vi "Set count lmits.vi"(8 "error in (no error)":errorcluster, 9 "Production max limit":dbl, 10 "Reel max limit":dbl, 11 "Counts":refnum<vi>) -> (0 "error out":errorcluster)   [LabVIEW 2019, in "ZenGage v3.0 UI.lvclass"]
uses:
  ZenGage v3.0 UI.lvclass
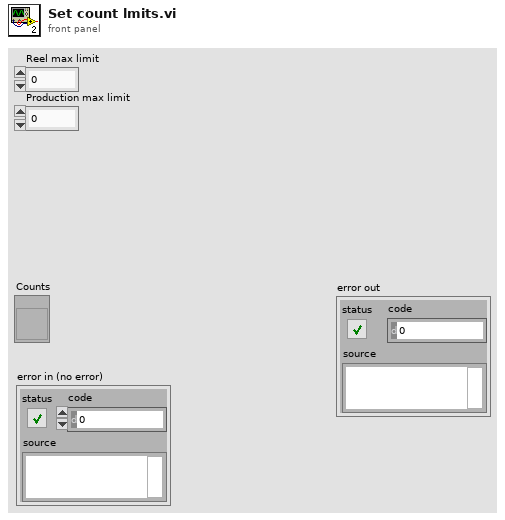
[diagram p1: front panel]
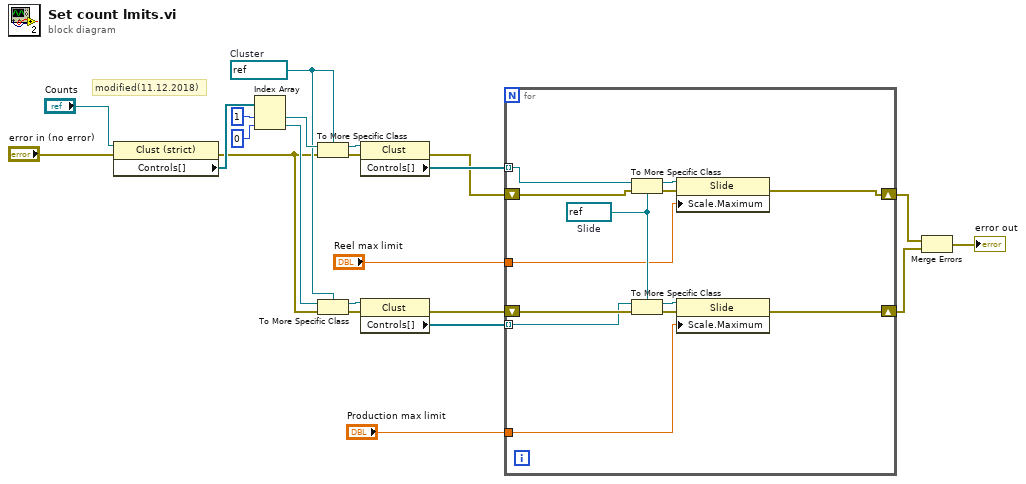
[diagram p0: block diagram]
diagram:
  w15 = refnum<vi> refnum  # Cluster
  # "modified(11.12.2018)"
  n1 = property class="Clust (strict)"(reference="Counts", error in="error in (no error)") -> (error out=w9:errorcluster, "Controls[]"=w22:refnum<vi>[])  [unwired: 1 out]
  n2 = Index Array(array=w22, index #1=1 ("index"), index #2=0 ("index")) -> (element #1=w19:refnum<vi>, element #2=w16:refnum<vi>)
  n3 = To More Specific Class(target class=w15, reference=w19, error in=w9) -> (specific class reference=w18:refnum<vi>, error out=w8:errorcluster)
  n4 = To More Specific Class(target class=w15, reference=w16, error in=w9) -> (specific class reference=w14:refnum<vi>, error out=w7:errorcluster)
  n5 = property class="Clust"(reference=w18, error in=w8) -> (error out=w6:errorcluster, "Controls[]"=w17:refnum<vi>[])  [unwired: 1 out]
  n6 = property class="Clust"(reference=w14, error in=w7) -> (error out=w5:errorcluster, "Controls[]"=w13:refnum<vi>[])  [unwired: 1 out]
  n7 = for {
    tunnel: w17 -> [w24] mode=indexing
    tunnel: w13 -> [w23] mode=indexing
    tunnel: "Reel max limit" -> [w32]
    tunnel: "Production max limit" -> [w31]
    shift-right: [w26] -> w2
    shift-left: w6 -> [w30]
    shift-right: [w25] -> w3
    shift-left: w5 -> [w29]
    w33 = refnum<vi> refnum  # Slide
    n8 = To More Specific Class(target class=w33, reference=w24, error in=w30) -> (specific class reference=w35:refnum<vi>, error out=w28:errorcluster)
    n9 = To More Specific Class(target class=w33, reference=w23, error in=w29) -> (specific class reference=w34:refnum<vi>, error out=w27:errorcluster)
    n10 = property class="Slide"(reference=w35, error in=w28, "Scale.Maximum"=w32) -> (error out=w26:errorcluster)  [unwired: 1 out]
    n11 = property class="Slide"(reference=w34, error in=w27, "Scale.Maximum"=w31) -> (error out=w25:errorcluster)  [unwired: 1 out]
  }
  n12 = Merge Errors(w2, w3) -> (→"error out":errorcluster)
